vi "Initialize Grating.vi"(8 "error in (no error)":errorcluster, 11 "VISA resource name":refnum<visa-resource-name>) -> (0 "error out":errorcluster, 3 "VISA resource name out":refnum<visa-resource-name>)   [LabVIEW 2017, in "JY-SPEX-TRIAX.lvlib"]
doc: "This command is used to initialize the spectrometer, and normally only needs to be called once, when all the hardware is powered on and the spectrometer controller's software is started. It can take a minute or so to complete."
uses:
  JY-SPEX-TRIAX.lvlib
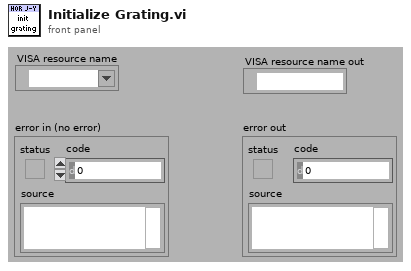
[diagram p1: front panel]
types:
  T1 = typedef "Semaphore RefNum" = refnum<k1>
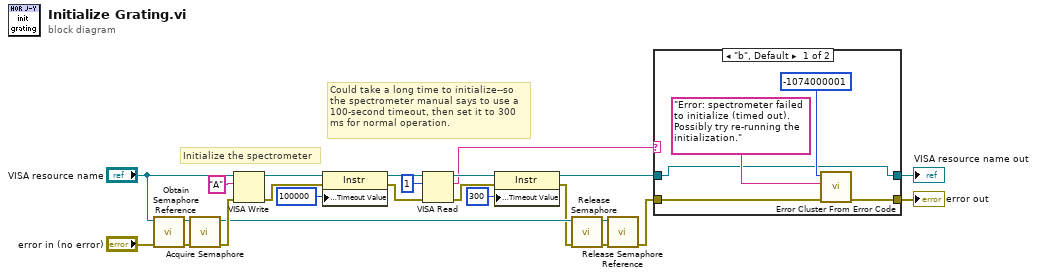
[diagram p0: block diagram]
diagram:
  # "Initialize the spectrometer"
  # "Could take a long time to initialize--so the spectrometer manual says to use a 100-second timeout, then set it to 300 ms for normal operation."
  n1 = call <vilib>:"Obtain Semaphore Reference.vi"("error in (no error)"="error in (no error)", "name (unnamed)"="VISA resource name") -> ("error out"=w10:errorcluster, "semaphore"=w9:T1)  [unwired: 1 in, 3 out]
  n2 = call <vilib>:"Acquire Semaphore.vi"("error in (no error)"=w10, "semaphore"=w9) -> ("error out"=w8:errorcluster, "semaphore out"=w3:T1)  [unwired: 1 in, 3 out]
  n3 = VISA Write(VISA resource name="VISA resource name", write buffer="A", error in (no error)=w8) -> (VISA resource name out=w22:refnum<visa-resource-name>, error out=w21:errorcluster)  [unwired: 1 out]
  n4 = property class="Instr"(reference=w22, error in=w21, "General Settings:Timeout Value"=u32 100000) -> (reference out=w20:refnum<visa-resource-name>, error out=w19:errorcluster)
  n5 = VISA Read(VISA resource name=w20, byte count=u32 1, error in (no error)=w19) -> (VISA resource name out=w16:refnum<visa-resource-name>, read buffer=w13:string, error out=w15:errorcluster)  [unwired: 1 out]
  n6 = property class="Instr"(reference=w16, error in=w15, "General Settings:Timeout Value"=u32 300) -> (reference out=w14:refnum<visa-resource-name>, error out=w2:errorcluster)
  n7 = call <vilib>:"Release Semaphore.vi"("error in (no error)"=w2, "semaphore"=w3) -> ("error out"=w5:errorcluster, "semaphore out"=w4:T1)  [unwired: 4 out]
  n8 = call <vilib>:"Release Semaphore Reference.vi"("error in (no error)"=w5, "semaphore"=w4) -> ("error out"=w1:errorcluster)  [unwired: 9 out]
  n9 = case shown="\"b\", Default" w13 {
    tunnel: w1 -> [w27 w30]
    tunnel: [w26 w30] -> w11
    tunnel: w14 -> [w25 w31]
    tunnel: [w25 w31] -> w12
    frame "b", Default {
      n10 = call <vilib>:"Error Cluster From Error Code.vi"("error in (no error)"=w27, "error message (\"\")"="Error: spectrometer failed to initialize (timed out).  Possibly try re-running the initialization." ("error message (\"\")"), "error code (0)"=-1074000001) -> ("error out"=w26:errorcluster)  [unwired: 1 in, 5 out]
    }
    frame "o" {
    }
  }
  "VISA resource name out" <- w12
  "error out" <- w11
